vi "Set String Variable.vi"(7 "Path":string, 8 "error in (no error)":errorcluster, 9 "Data":string, 11 "JSON Variable in":refnum<class "JSON Variable.lvclass">) -> (0 "error out":errorcluster, 3 "JSON Variable out":refnum<class "JSON Variable.lvclass">)   [LabVIEW 2019, in "JSON Variable.lvclass"]
uses:
  JSON Variable.lvclass
  c38bf80d-fa51-4496-ad5b-fb621cb4c5f3.vi
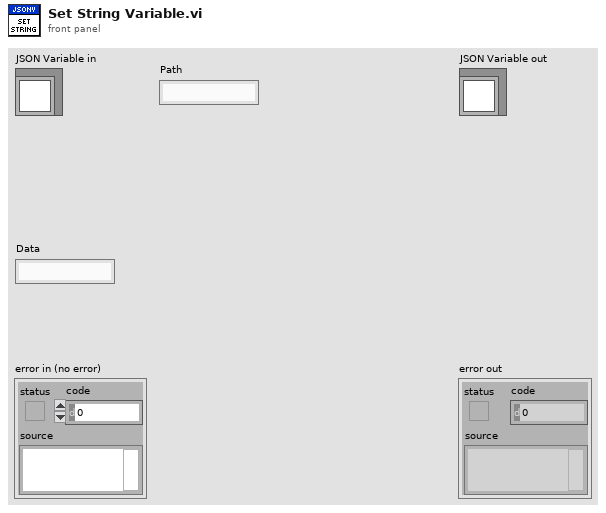
[diagram p1: front panel]
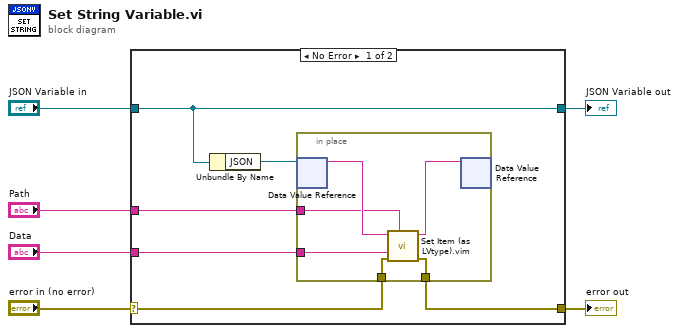
[diagram p0: block diagram]
diagram:
  n1 = case shown="No Error" "error in (no error)" {
    selector: "error in (no error)" -> [w8 w20]
    tunnel: [w7 w20] -> w5
    tunnel: [w12 w19] -> w3
    tunnel: "JSON Variable in" -> [w12 w19]
    tunnel: "Path" -> [w10 _]
    tunnel: "Data" -> [w9 _]
    frame No Error {
      n2 = Unbundle By Name(w12) -> ("JSON"=w11:refnum<data-value>)
      n3 = in-place {
        in-place-border: w10 -> [w17]
        in-place-border: w9 -> [w16]
        in-place-border: w8 -> [w15]
        in-place-border: [w14] -> w7
        n4 = in-place-dvr #1(w11) -> (w18:string)  [unwired: 1 out]
        n5 = call "Set Item (as LVtype).vim"("Object (or Item) Path"=w17, "error in (no error)"=w15, "Anything"=w16, "JSON"=w18) -> ("error out"=w14:errorcluster, "<JSON>"=w13:string)  [unwired: 4 in, 1 out]
        n6 = in-place-dvr #1(w13) -> ()  [unwired: 2 out]
      }
    }
    frame Error {
    }
  }
  "error out" <- w5
  "JSON Variable out" <- w3
